vi "SCD Acquisition.vi"(8 "error in (no error)":errorcluster) -> (0 "error out":errorcluster)   [LabVIEW 2023, in "Examples.lvlib"]
uses:
  Examples.lvlib
  Classes/SCD/SCD.lvclass
  Classes/SCD/acqSet.ctl
  09379220-ee7b-4c62-9ded-10c8c6150607.vi
  d2e59c47-dc5d-4a76-9504-18b862921f36.vi
panel:
  out "data":T1(array[cluster])
  out "isDataAvailable?":bool
  out "isBusy":bool
  # "Connector Pane"
  # "Locals"
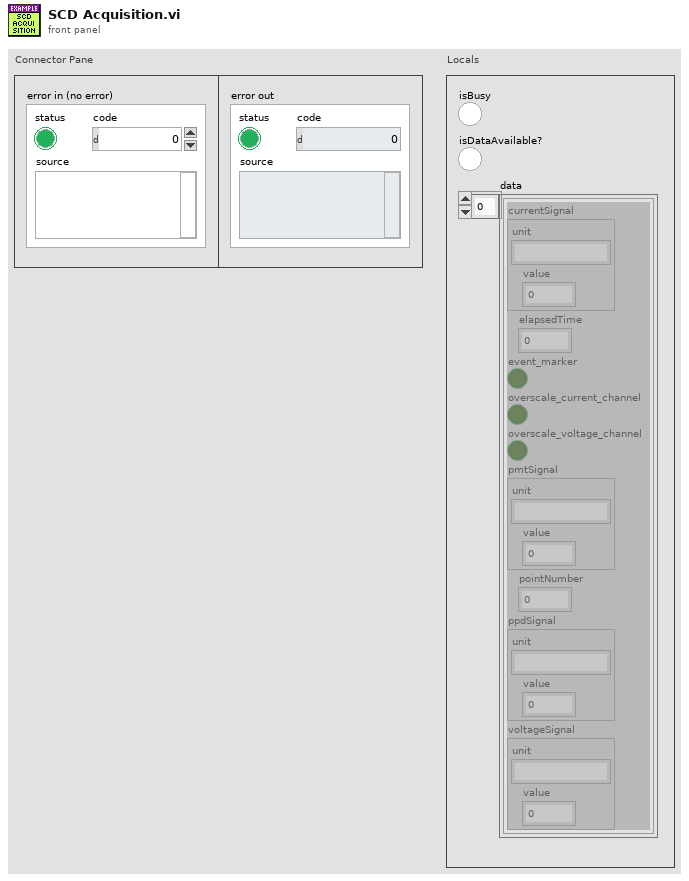
[diagram p1: front panel]
types:
  T1 = cluster{"currentSignal":cluster{"unit":string, "value":dbl}, "elapsedTime":dbl, "event_marker":bool, "overscale_current_channel":bool, "overscale_voltage_channel":bool, "pmtSignal":cluster{"unit":string, "value":dbl}, "pointNumber":dbl, "ppdSignal":cluster{"unit":string, "value":dbl}, "voltageSignal":cluster{"unit":string, "value":dbl}}[]
  T2 = typedef "horiba.lvlib/SCD.lvclass/acqSet.ctl" = cluster{"scanCount":i32, "timeStep":i32, "integrationTime":i32, "externalParam":i32}
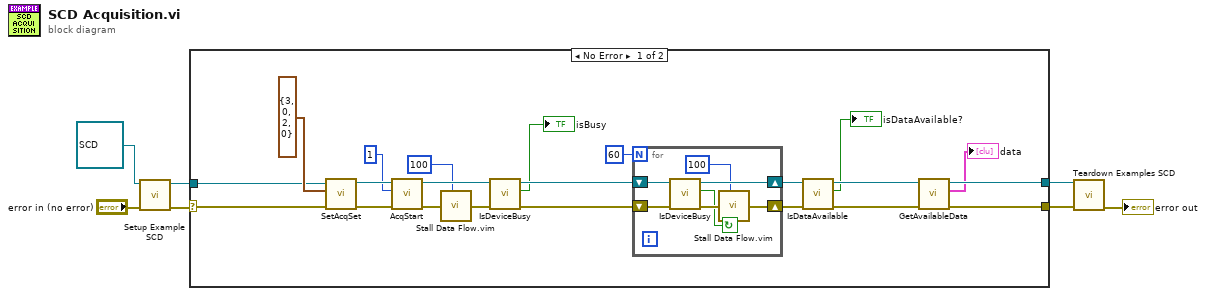
[diagram p0: block diagram]
diagram:
  n1 = call "Setup Example SCD.vi"("error in (no error)"="error in (no error)", "SCD in"=refnum<class "SCD.lvclass"> refnum) -> ("error out"=w4:errorcluster, "SCD out"=w3:refnum<class "SCD.lvclass">)  [unwired: 6 in, 2 out]
  n2 = case shown="No Error" w4 {
    selector: w4 -> [w29 w38]
    tunnel: [w17 w37] -> w2
    tunnel: [w19 w38] -> w1
    tunnel: w3 -> [w12 w37]
    frame No Error {
      n3 = call "SetAcqSet.vi"("error in (no error)"=w29, "integration_time"=T2 {"scanCount"=3, "timeStep"=0, "integrationTime"=2, "externalParam"=0}, "SCD in"=w12) -> ("error out"=w28:errorcluster, "SCD out"=w26:refnum<class "SCD.lvclass">)  [unwired: 7 in]
      n4 = call "AcqStart.vi"("error in (no error)"=w28, "trigger"=1, "SCD in"=w26) -> ("error out"=w27:errorcluster, "SCD out"=w24:refnum<class "SCD.lvclass">)  [unwired: 7 in]
      n5 = call "Stall Data Flow.vim"("value in"=w27, "milliseconds to wait"=u32 100) -> ("value out"=w23:errorcluster)  [unwired: 1 out]
      n6 = call "IsDeviceBusy.vi"("error in (no error)"=w23, "SCD in"=w24) -> ("error out"=w15:errorcluster, "isBusy"=→"isBusy":bool, "SCD out"=w20:refnum<class "SCD.lvclass">)  [unwired: 7 in]
      n7 = for {
        N: 60 -> [_]
        shift-right: [w35] -> w16
        shift-left: w20 -> [w36]
        shift-right: [w31] -> w14
        shift-left: w15 -> [w34]
        stop <- w32 continue-if-true
        n8 = call "IsDeviceBusy.vi"("error in (no error)"=w34, "SCD in"=w36) -> ("error out"=w33:errorcluster, "isBusy"=w32:bool, "SCD out"=w35:refnum<class "SCD.lvclass">)  [unwired: 7 in]
        n9 = call "Stall Data Flow.vim"("value in"=w33, "milliseconds to wait"=u32 100) -> ("value out"=w31:errorcluster)  [unwired: 1 out]
      }
      n10 = call "IsDataAvailable.vi"("error in (no error)"=w14, "SCD in"=w16) -> ("error out"=w21:errorcluster, "isDataAvailable?"=→"isDataAvailable?":bool, "SCD out"=w18:refnum<class "SCD.lvclass">)  [unwired: 7 in]
      n11 = call "GetAvailableData.vi"("error in (no error)"=w21, "SCD in"=w18) -> ("error out"=w19:errorcluster, "data"=→"data":T1, "SCD out"=w17:refnum<class "SCD.lvclass">)  [unwired: 7 in]
    }
    frame Error {
    }
  }
  n12 = call "Teardown Examples SCD.vi"("error in (no error)"=w1, "Monochromator in"=w2) -> ("error out"=→"error out":errorcluster)  [unwired: 9 in]
